vi "SmoothMoveSplitter.vi"(8 "error in (no error)":errorcluster, 9 "Steps (16)":i32=16, 10 "Position":i32, 11 "Splitter in":refnum<vi>) -> (0 "error out":errorcluster)   [LabVIEW 2012, in "Win8uiFramework.lvlib" / "MainController.lvclass"]
uses:
  MainController.lvclass
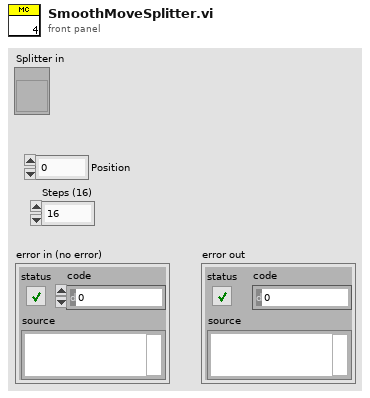
[diagram p1: front panel]
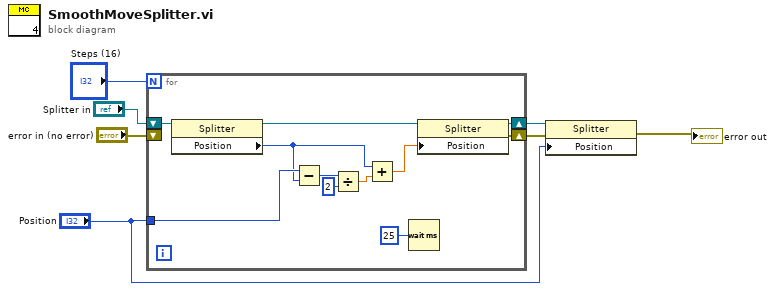
[diagram p0: block diagram]
diagram:
  n1 = for {
    N: "Steps (16)" -> [_]
    tunnel: "Position" -> [w15]
    shift-right: [w18] -> w3
    shift-left: "error in (no error)" -> [_]
    shift-right: [w9] -> w4
    shift-left: "Splitter in" -> [w17]
    n2 = property class="Splitter"(reference=w17) -> (reference out=w16:refnum<vi>, "Position"=w12:i32)  [unwired: 1 in, 1 out]
    n3 = Subtract(x=w15, y=w12) -> (x-y=w14:i32)
    n4 = Divide(x=w14, y=2) -> (x/y=w13:dbl)
    n5 = Add(x=w12, y=w13) -> (x+y=w11:dbl)
    n6 = Wait (ms)(milliseconds to wait=u32 25) -> ()  [unwired: 1 out]
    n7 = property class="Splitter"(reference=w16, "Position"=w11) -> (reference out=w9:refnum<vi>, error out=w18:errorcluster)  [unwired: 1 in]
  }
  n8 = property class="Splitter"(reference=w4, error in=w3, "Position"="Position") -> (error out=→"error out":errorcluster)  [unwired: 1 out]
